vi "Test Bench v16 - TDMS.vi"() -> ()   [LabVIEW 2022 SP3]
uses:
  WhiteNoise.ctl
  <vilib>/Utility/error.llb/DialogType.ctl
  <vilib>/Platform/TimedLoop/XDataNode/timing_clust.ctl
  <vilib>/Platform/TimedLoop/XDataNode/nitl_modes.ctl
  <vilib>/Platform/TimedLoop/XDataNode/wakeup.ctl
  <vilib>/DAQmx/write.llb/DAQmx Write (Analog 2D DBL NChan NSamp).vi
  <vilib>/DAQmx/read.llb/DAQmx Read (Analog 1D DBL 1Chan NSamp).vi
  <vilib>/DAQmx/create/channels.llb/DAQmx Create Channel (AI-Acceleration-Accelerometer).vi
  <vilib>/DAQmx/create/channels.llb/DAQmx Create Channel (AO-Voltage-Basic).vi
  <vilib>/DAQmx/configure/timing.llb/DAQmx Timing (Sample Clock).vi
  <vilib>/DAQmx/miscellaneous.llb/DAQmx Fill In Error Info.vi
  <vilib>/Platform/TimedLoop/TimeConversion.llb/rt-milliseconds-to-timestamp.vi
  <vilib>/Platform/TimedLoop/TimeConversion.llb/rt-milliseconds-to-rel-time.vi
  <vilib>/platform/TimedLoop/XDataNode/XDataNode.xnode
  <resource>/objmgr/daqmx.rc
  <vilib>/measure/NI_MABase.lvlib
  <vilib>/Platform/TimedLoop/XDataNode/XDNodeRunTimeDep.lvlib
panel:
  out "Actual Start [i]":timestamp
  out "Frame Duration":dbl
  out "TotalSampPerChanAcquired":dbl
  out "Actual End [f-1]":timestamp
  in  "stop":bool
  out "SampClk.Rate":dbl
  out "Accel. 1 Raw":dbl[](graph)
  in  "Enable Display":bool=TRUE
  in  "Folder to save file to":path=path "C:/Users/LAV-UFSC-2023/Documents/LAV-TCC/Dados-Experimentos/Dados-Bancada-LABVIEW"
  out "Output Signal":dynamicdata(graph)
  in  "Accel. 2":bool
  out "New file path":path
  in  "Signal Output\nControl":enum32{"White Noise", "Harmonic"}(tab)
  in  "White Noise\nParameters":T2={"Seed"=0.0, "Standard Deviation"=0.2, "Reset"=FALSE, "Iterator"=1.0, "Seed"=-1, "Lower Cut-Off"=5.0, "Upper Cut-Off"=350.0} {"Upper Cut-Off" min=5.0 max=350.0 step=10.0; "Lower Cut-Off" min=5.0 max=350.0 step=10.0; "Standard Deviation" min=0.001 max=3.0 step=0.05 format="%0.2p"}
  out "dt White Noise":dbl
  in  "Hamonic\nParameters":T3={"Waveform Type"=0, "Frequency"=10.0, "Amplitude"=0.25} {"Frequency" min=5.0 max=350.0 step=10.0 format="%0.2p"; "Waveform Type" items=["Sine Wave", "Triangle Wave", "Square Wave", "Sawtooth Wave"]; "Amplitude" min=0.001 max=0.3 step=0.05 format="%0.2p"}
  out "dt Harmonic":dbl
  in  "Output":bool=TRUE
  # "Filter"
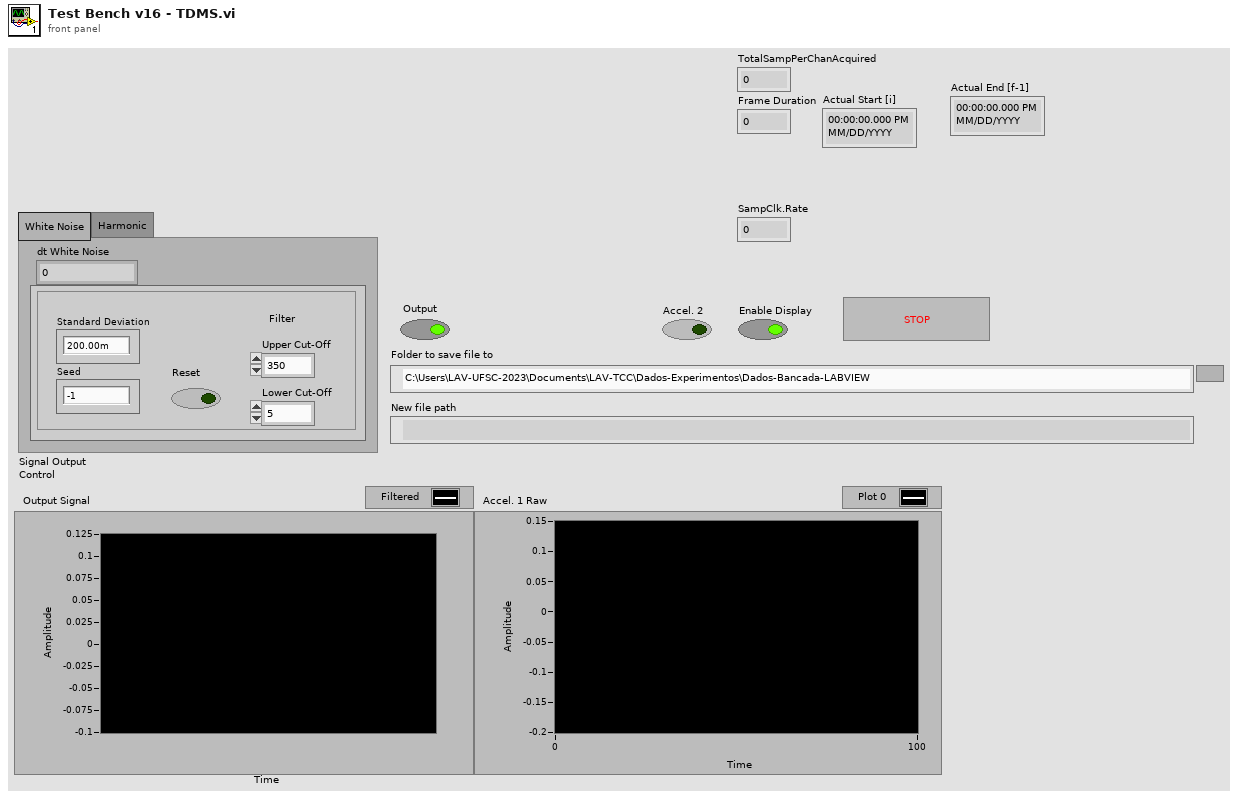
[diagram p1: front panel]
types:
  T1 = typedef "WhiteNoise.ctl" = dbl
  T2 = cluster{"Seed":T1, "Standard Deviation":dbl, "Reset":bool, "Iterator":dbl, "Seed":i8, "Lower Cut-Off":dbl, "Upper Cut-Off":dbl}
  T3 = cluster{"Waveform Type":u16, "Frequency":dbl, "Amplitude":dbl}
  T4 = typedef "DialogType.ctl" = u16
  T5 = enum16{"open", "open or create", "create or replace", "create", "open (read-only)"}
  T6 = typedef "XDNodeRunTimeDep.lvlib/timing_clust.ctl" = cluster{"Expected End [f-1]":u64, "Actual End [f-1]":u64, "Finished Late? [f-1]":bool, "Expected End [i-1]":u64, "Actual End [i-1]":u64, "Finished Late? [i-1]":bool, "Expected Start [i]":u64, "Actual Start [i]":u64, "Expected Start [f]":u64, "Actual Start [f]":u64, "Source Name":string, "Structure Name":string, "Period":i64, "Deadline":i64, "Offset":i64, "Start":i64, "Priority":i32, "Timeout":i32, "Mode":T7, "Wakeup Reason":T8, "Error":errorcluster, "Source Type":string, "Secondary Source Type":string, "Global End Time":u64, "Global Start Time":u64, "Frame Duration":u64, "Iteration Duration":u64, "Assigned CPU":i32, "I/O Scan Engine Mode":u32}
  T7 = typedef "XDNodeRunTimeDep.lvlib/nitl_modes.ctl" = enum32{"No Change", "Process missed periods, maintain original phase", "Discard missed periods, maintain original phase", "Process missed periods, ignore original phase", "Discard missed periods, ignore original phase"}
  T8 = typedef "XDNodeRunTimeDep.lvlib/wakeup.ctl" = enum32{"Normal", "Aborted", "Asynchronous wakeup", "Timing source error", "Timed loop error", "Timeout"}
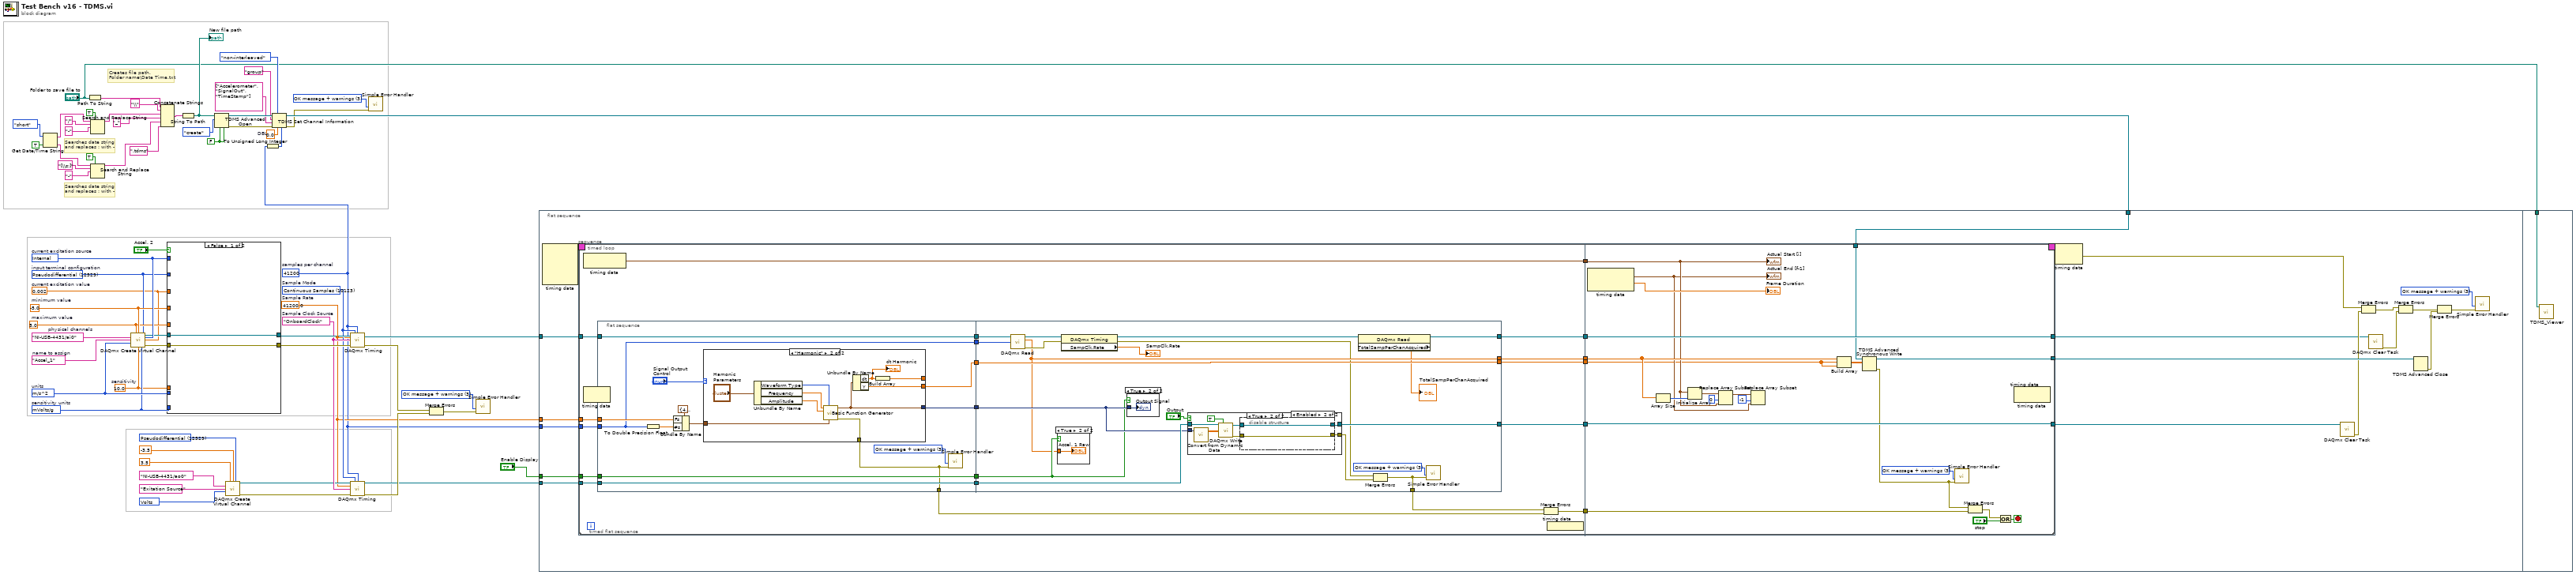
[diagram p0: block diagram]
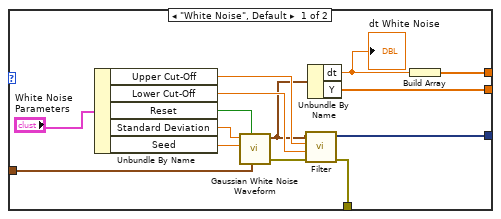
[diagram p2: hidden frame]
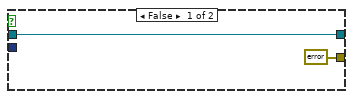
[diagram p5: hidden frame]
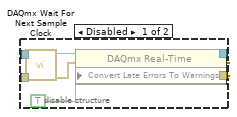
[diagram p6: hidden frame]
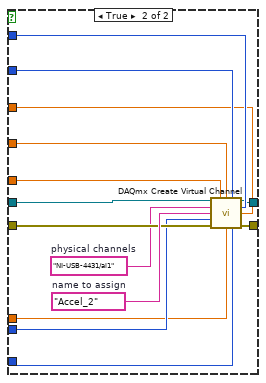
[diagram p7: hidden frame]
diagram:
  w6 = T4 3 items=["no dialog", "OK message", "continue or stop message", "OK message + warnings", "continue/stop + warnings"] ("type of dialog (OK msg:1)")
  w1 = 41200  # samples per channel
  w10 = 0.0  # DBL
  w12 = FALSE ("enable asynchronous? (T)")
  w8 = T4 3 items=["no dialog", "OK message", "continue or stop message", "OK message + warnings", "continue/stop + warnings"] ("type of dialog (OK msg:1)")
  w52 = 12529 items=["Default"=-1, "RSE"=10083, "Differential"=10106, "Pseudodifferential"=12529] ("output terminal configuration")
  w50 = 10348 items=["Volts"=10348, "From Custom Scale"=10065] ("units")
  w56 = 12509 items=["mVolts/g"=12509, "Volts/g"=12510]  # sensitivity units
  w47 = 10.0  # sensitivity
  w55 = 0.002  # current excitation value
  w63 = 10200 items=["Internal"=10200, "External"=10167, "None"=10230]  # current excitation source
  w57 = tag "NI-USB-4431/ai0"  # physical channels
  w44 = tag "OnboardClock"  # Sample Clock Source
  w3 = 41200.0  # Sample Rate
  w43 = 10123 items=["Finite Samples"=10178, "Continuous Samples"=10123, "Hardware Timed Single Point"=12522]  # Sample Mode
  w59 = 12529 items=["default"=-1, "RSE"=10083, "NRSE"=10078, "Differential"=10106, "Pseudodifferential"=12529]  # input terminal configuration
  w62 = -5.0  # minimum value
  w61 = 5.0  # maximum value
  w65 = "Accel_1"  # name to assign
  w60 = 12470 items=["g"=10186, "m/s^2"=12470, "in/s^2"=12471, "From Custom Scale"=10065]  # units
  # "Searches date string\nand replaces : with -"
  # "Searches date string\nand replaces : with -"
  # "Creates file path.\nFolder name\\Date Time.txt"
  n1 = Get Date/Time String(date format (0)=enum16{"short", "long", "abbreviated"}."short", want seconds? (F)=TRUE) -> (date string=w20:string, time string=w33:string)  [unwired: 1 in]
  n2 = Path To String(path="Folder to save file to") -> (string=w28:string)
  n3 = Search and Replace String(replace all?=TRUE ("replace all? (F)"), input string=w20, search string="/" ("replace string (\"\")"), replace string="-" ("replace string (\"\")")) -> (result string=w19:string)  [unwired: 4 in, 3 out]
  n4 = Search and Replace String(replace all?=TRUE ("replace all? (F)"), input string=w33, search string="[\\s:]" ("replace string (\"\")"), replace string="-" ("replace string (\"\")")) -> (result string=w26:string)  [unwired: 4 in, 3 out]
  n5 = call-poly <vilib>:"DAQmx Create Virtual Channel.vi"("maximum value"=w61, "minimum value"=w62, "input terminal configuration"=w59, "physical channels"=w57, "current excitation source"=w63, "name to assign"=w65, "current excitation value"=w55, "units"=w60, "sensitivity"=w47, "sensitivity units"=w56) -> ("task out"=w58:refnum<k21>, "error out"=w64:errorcluster)  [unwired: 4 in]
  n6 = Concatenate Strings(w28, "\\" ("string"), w19, "_" ("string"), w26, ".tdms" ("string")) -> (w24:string)
  n7 = case shown="False" "Accel. 2" {
    tunnel: w64 -> [w67 w80]
    tunnel: w63 -> [_ w79]
    tunnel: w62 -> [_ w78]
    tunnel: w61 -> [_ w77]
    tunnel: w60 -> [_ w76]
    tunnel: w59 -> [_ w75]
    tunnel: w58 -> [w66 w74]
    tunnel: w56 -> [_ w72]
    tunnel: w55 -> [_ w71]
    tunnel: w47 -> [_ w70]
    tunnel: [w67 w69] -> w46
    tunnel: [w66 w68] -> w45
    frame False {
    }
    frame True {
      w73 = tag "NI-USB-4431/ai1"  # physical channels
      w81 = "Accel_2"  # name to assign
      n8 = call-poly <vilib>:"DAQmx Create Virtual Channel.vi"("task in"=w74, "maximum value"=w77, "minimum value"=w78, "input terminal configuration"=w75, "physical channels"=w73, "current excitation source"=w79, "name to assign"=w81, "current excitation value"=w71, "units"=w76, "error in"=w80, "sensitivity"=w70, "sensitivity units"=w72) -> ("task out"=w68:refnum<k21>, "error out"=w69:errorcluster)  [unwired: 2 in]
    }
  }
  n9 = String To Path(string=w24) -> (path=w37:path)
  "New file path" <- w37
  n10 = TDMS Advanced Open(4:w12, 6:w12, 10:T5."create" ("operation (0:open)"), 11:w37) -> (0:w16:errorcluster, 3:w15:refnum<k34>)  [unwired: 1 in, 1 out]
  n11 = call-poly <vilib>:"DAQmx Create Virtual Channel.vi"("maximum value"=3.5, "minimum value"=-3.5, "output terminal configuration"=w52, "physical channels"=tag "NI-USB-4431/ao0", "name to assign"="Exitation Source", "units"=w50) -> ("task out"=w41:refnum<k21>, "error out"=w42:errorcluster)  [unwired: 8 in]
  n12 = To Unsigned Long Integer(number=w1) -> (unsigned 32bit integer=w2:u32)
  n13 = TDMS Set Channel Information(4:w2, 6:w10, 7:enum16{"non-interleaved", "interleaved"}."non-interleaved" ("data layout (0:non-interleaved)"), 8:w16, 9:string[] ["Accelerometer", "SignalOut", "TimeStamp"] ("channel name(s)"), 10:"group" ("group name (Untitled)"), 11:w15) -> (0:w9:errorcluster, 3:w36:refnum<k34>)
  n14 = call-poly <vilib>:"DAQmx Timing.vi"("task/channels in"=w45, "sample mode"=w43, "samples per channel"=w1, "rate"=w3, "source"=w44, "error in"=w46) -> ("task out"=w5:refnum<k21>, "error out"=w49:errorcluster)  [unwired: 8 in]
  n15 = call-poly <vilib>:"DAQmx Timing.vi"("task/channels in"=w41, "sample mode"=w43, "samples per channel"=w1, "rate"=w3, "source"=w44, "error in"=w42) -> ("task out"=w39:refnum<k21>, "error out"=w40:errorcluster)  [unwired: 8 in]
  n16 = call <vilib>:"Simple Error Handler.vi"("type of dialog (OK msg:1)"=w8, "error in (no error)"=w9) -> ()  [unwired: 3 in, 5 out]
  n17 = Merge Errors(w49, w40) -> (w4:errorcluster)
  n18 = call <vilib>:"Simple Error Handler.vi"("type of dialog (OK msg:1)"=w6, "error in (no error)"=w4) -> ()  [unwired: 3 in, 5 out]
  n19 = flat-sequence {
    tunnel: w39 -> [w97]
    tunnel: w5 -> [w95]
    tunnel: w36 -> [w84]
    tunnel: "Enable Display" -> [w93]
    tunnel: w3 -> [w83]
    tunnel: w1 -> [w82]
    tunnel: "Folder to save file to" -> [w257]
    frame #0 {
      w98 = T4 3 items=["no dialog", "OK message", "continue or stop message", "OK message + warnings", "continue/stop + warnings"] ("type of dialog (OK msg:1)")
      n20 = node-c288() -> (w100:T6)  [unwired: 4 in]
      n21 = timed-loop {
        tunnel: w97 -> [w109]
        tunnel: [w108] -> w96
        tunnel: w95 -> [w107]
        tunnel: [w103] -> w90
        tunnel: [w102] -> w94
        tunnel: w93 -> [w106]
        tunnel: w82 -> [w105]
        timing: w100 -> [_]
        timing-out: [_] -> w99
        tunnel: w84 -> [w104]
        tunnel: w83 -> [w101]
        stop <- w241 stop-if-true
        n22 = timed-sequence {
          timing: _ -> [_]
          timing-out: _ -> [_]
          tunnel: w109 -> [w124]
          tunnel: [w123] -> w108
          tunnel: w107 -> [w122]
          tunnel: w106 -> [w121]
          tunnel: w105 -> [w120]
          tunnel: w104 -> [w116]
          tunnel: [w115] -> w103
          tunnel: [w112] -> w102
          tunnel: w101 -> [w110]
          n23 = timed-flat-sequence {
            tunnel: w124 -> [w137]
            tunnel: w122 -> [w136]
            tunnel: w121 -> [w133]
            tunnel: w120 -> [w132]
            tunnel: [w135] -> w119
            tunnel: [w134] -> w118
            tunnel: [w129] -> w117
            tunnel: [w128] -> w114
            tunnel: [w127] -> w113
            tunnel: [w126] -> w111
            tunnel: w110 -> [w125]
            tunnel: [w245] -> w123
            tunnel: w119 -> [w245]
            tunnel: w118 -> [w238]
            tunnel: w117 -> [w242]
            tunnel: w116 -> [w236]
            tunnel: [w238] -> w115
            tunnel: w114 -> [w231]
            tunnel: w113 -> [w225]
            tunnel: [w235] -> w112
            tunnel: w111 -> [w229]
            frame #0 {
              n24 = node-c288() -> (w126:timestamp)  [unwired: 1 in]
              n25 = flat-sequence {
                tunnel: [w157] -> w143
                tunnel: [w153] -> w142
                tunnel: [w156] -> w141
                tunnel: [w154] -> w140
                tunnel: [w155] -> w139
                tunnel: [w149] -> w138
                tunnel: [w152] -> w130
                tunnel: w137 -> [w156]
                tunnel: w136 -> [w157]
                tunnel: w133 -> [w154]
                tunnel: w132 -> [w149]
                tunnel: w125 -> [w150]
                tunnel: w143 -> [w195]
                tunnel: w142 -> [w203]
                tunnel: w141 -> [w201]
                tunnel: w140 -> [w196]
                tunnel: w139 -> [w199]
                tunnel: w138 -> [w194]
                tunnel: [w188] -> w131
                tunnel: [w192] -> w128
                tunnel: [w203] -> w127
                tunnel: [w200] -> w135
                tunnel: [w187] -> w134
                frame #0 {
                  w151 = T4 3 items=["no dialog", "OK message", "continue or stop message", "OK message + warnings", "continue/stop + warnings"] ("type of dialog (OK msg:1)")
                  n26 = To Double Precision Float(number=w149) -> (double precision float=w148:dbl)
                  n27 = Bundle By Name(cluster=cluster{"Fs":dbl, "#s":dbl} {"Fs"=41200.0, "#s"=41200.0} ("sampling info"), "Fs"=w150, "#s"=w148) -> (w159:cluster{"Fs":dbl, "#s":dbl})
                  n28 = case shown="\"Harmonic\"" "Signal Output\nControl" {
                    tunnel: w159 -> [w172 w183]
                    tunnel: [w164 w178] -> _
                    tunnel: [w163 w177] -> w155
                    tunnel: [w162 w176] -> w153
                    tunnel: [w161 w175] -> w152
                    frame "White Noise", Default {
                      n29 = Unbundle By Name("White Noise\nParameters") -> ("Upper Cut-Off"=w168:dbl, "Lower Cut-Off"=w167:dbl, "Reset"=w169:bool, "Standard Deviation"=w170:dbl, "Seed"=w171:T1)
                      n30 = call <vilib>:"Gaussian White Noise Waveform.vi"("sampling info"=w172, "reset signal"=w169, "seed"=w171, "standard deviation"=w170) -> ("error out"=w174:errorcluster, "signal out"=w166:waveform(dbl))  [unwired: 6 in]
                      n31 = call "Filter"("error in (no error)"=w174, "Lower Cut-Off"=w167, "Upper Cut-Off"=w168, "Signal"=w166) -> ("error out"=w161:errorcluster, "Filtered Signal"=w163:dynamicdata)  [unwired: 6 in]
                      n32 = Unbundle By Name(w166) -> ("dt"=w165:dbl, "Y"=w162:dbl[])
                      "dt White Noise" <- w165
                      n33 = Build Array(w165) -> (w164:dbl[])
                    }
                    frame "Harmonic" {
                      n34 = Unbundle By Name("Hamonic\nParameters") -> ("Waveform Type"=w182:u16, "Frequency"=w181:dbl, "Amplitude"=w180:dbl)
                      n35 = call <vilib>:"Basic Function Generator.vi"("sampling info"=w183, "signal type"=w182, "amplitude"=w180, "frequency"=w181) -> ("error out"=w175:errorcluster, "signal out"=w177:waveform(dbl))  [unwired: 5 in, 1 out]
                      n36 = Unbundle By Name(w177) -> ("dt"=w179:dbl, "Y"=w176:dbl[])
                      "dt Harmonic" <- w179
                      n37 = Build Array(w179) -> (w178:dbl[])
                    }
                  }
                  n38 = call <vilib>:"Simple Error Handler.vi"("type of dialog (OK msg:1)"=w151, "error in (no error)"=w152) -> ()  [unwired: 3 in, 5 out]
                }
                frame #1 {
                  w191 = T4 3 items=["no dialog", "OK message", "continue or stop message", "OK message + warnings", "continue/stop + warnings"] ("type of dialog (OK msg:1)")
                  n39 = call-poly <vilib>:"DAQmx Read.vi"("task/channels in"=w195, "number of samples per channel"=w194) -> ("task out"=w197:refnum<k21>, "data"=w192:dbl[], "error out"=w198:errorcluster)  [unwired: 11 in]
                  n40 = case shown="True" w196 {
                    tunnel: w192 -> [_ w204]
                    frame False {
                    }
                    frame True {
                      "Accel. 1 Raw" <- w204
                    }
                  }
                  n41 = property class="DAQmx Timing"(reference=w197, error in=w198) -> (reference out=w186:refnum<k21>, error out=w190:errorcluster, "SampClk.Rate"=→"SampClk.Rate":dbl)
                  n42 = case shown="True" w196 {
                    tunnel: w199 -> [_ w205]
                    frame False {
                    }
                    frame True {
                      "Output Signal" <- w205
                    }
                  }
                  n43 = case shown="True" "Output" {
                    tunnel: w201 -> [w207 w215]
                    tunnel: [errorcluster {"status"=FALSE, "code"=0, "source"=""} ("error out") w211] -> w189
                    tunnel: [w207 w212] -> w200
                    tunnel: w199 -> [_ w210]
                    frame False {
                    }
                    frame True {
                      n44 = call "Convert from Dynamic Data"("Dynamic Data Type"=w210) -> ("Array"=w209:dbl[][])  [unwired: 3 in]
                      n45 = call-poly <vilib>:"DAQmx Write.vi"("task/channels in"=w215, "auto start"=TRUE, "data"=w209) -> ("task out"=w214:refnum<k21>, "error out"=w213:errorcluster)  [unwired: 10 in, 1 out]
                      n46 = disable-structure shown="Enabled" {
                        disable-tunnel: w214 -> [w222 w223]
                        disable-tunnel: w213 -> [w221 w224]
                        disable-tunnel: [w219 w223] -> w212
                        disable-tunnel: [w218 w224] -> w211
                        frame Disabled {
                          n47 = call <vilib>:"DAQmx Wait For Next Sample Clock.vi"("task/channels in"=w222, "error in"=w221) -> ("task out"=w220:refnum<k21>, "error out"=w217:errorcluster)  [unwired: 11 in, 1 out]
                          n48 = property class="DAQmx Real-Time"(reference=w220, error in=w217, "Convert Late Errors To Warnings"=TRUE ("ConvLateErrorsToWarnings")) -> (reference out=w219:refnum<k21>, error out=w218:errorcluster)
                        }
                        frame Enabled {
                        }
                      }
                    }
                  }
                  n49 = property class="DAQmx Read"(reference=w186) -> (reference out=w187:refnum<k21>, "TotalSampPerChanAcquired"=→"TotalSampPerChanAcquired":dbl)  [unwired: 1 in, 1 out]
                  n50 = Merge Errors(w190, w189) -> (w188:errorcluster)
                  n51 = call <vilib>:"Simple Error Handler.vi"("type of dialog (OK msg:1)"=w191, "error in (no error)"=w188) -> ()  [unwired: 3 in, 5 out]
                }
              }
              n52 = Merge Errors(w131, w130) -> (w129:errorcluster)
              n53 = node-c288() -> ()  [unwired: 1 out]
            }
            frame #1 {
              w239 = T4 3 items=["no dialog", "OK message", "continue or stop message", "OK message + warnings", "continue/stop + warnings"] ("type of dialog (OK msg:1)")
              n54 = node-c288() -> (w226:timestamp, →"Frame Duration":dbl)  [unwired: 1 in]
              "Actual End [f-1]" <- w226
              n55 = Array Size(array=w231) -> (size(s)=w232:i32)
              n56 = Initialize Array(w229, w232) -> (w233:timestamp[])
              n57 = Replace Array Subset(array=w233, new element=w229, index=0) -> (w227:timestamp[])
              n58 = Replace Array Subset(array=w227, new element=w226, index=-1) -> ()  [unwired: 1 out]
              n59 = Build Array(w231, w225, w225) -> (w240:dbl[][])
              n60 = TDMS Advanced Synchronous Write(10:w240, 11:w236) -> (0:w237:errorcluster, 3:w235:refnum<k34>)  [unwired: 1 in]
              n61 = call <vilib>:"Simple Error Handler.vi"("type of dialog (OK msg:1)"=w239, "error in (no error)"=w237) -> ()  [unwired: 3 in, 5 out]
              n62 = Merge Errors(w237, w242) -> (w244:errorcluster)
              n63 = Or(x=w244, y="stop") -> (x .or. y?=w241:bool)
              n64 = node-c288() -> ()  [unwired: 1 in, 1 out]
              "Actual Start [i]" <- w229
            }
          }
        }
        n65 = node-c288() -> ()  [unwired: 1 in, 1 out]
        n66 = node-c288() -> ()  [unwired: 1 in, 1 out]
      }
      n67 = node-c288(w99) -> (w85:errorcluster)
      n68 = call <vilib>:"DAQmx Clear Task.vi"("task in"=w96) -> ("error out"=w92:errorcluster)  [unwired: 14 in]
      n69 = Merge Errors(w85, w92) -> (w89:errorcluster)
      n70 = call <vilib>:"DAQmx Clear Task.vi"("task in"=w90) -> ("error out"=w88:errorcluster)  [unwired: 14 in]
      n71 = Merge Errors(w89, w88) -> (w87:errorcluster)
      n72 = TDMS Advanced Close(11:w94) -> (0:w91:errorcluster)  [unwired: 3 in, 1 out]
      n73 = Merge Errors(w87, w91) -> (w86:errorcluster)
      n74 = call <vilib>:"Simple Error Handler.vi"("type of dialog (OK msg:1)"=w98, "error in (no error)"=w86) -> ()  [unwired: 3 in, 5 out]
    }
    frame #1 {
      n75 = call "TDMS_Viewer.vi"("Data Directory"=w257) -> ()  [unwired: 11 in]
    }
  }
